vi "TestStand RunState Fields.vi"(2 "index":i32) -> (14 "Measurement Name":string, 15 "Low Limit":string, 16 "High Limit":string, 17 "Units":string, 18 "Comp":string, 19 "Data":string)   [LabVIEW 2010]
doc: "Creates strings with TestStand Numeric Test Property Names."
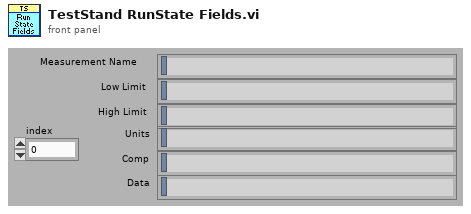
[diagram p1: front panel]
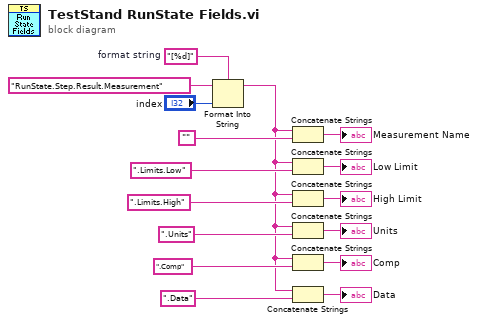
[diagram p0: block diagram]
diagram:
  w8 = "[%d]"  # format string
  n1 = Format Into String(format string=w8, initial string="RunState.Step.Result.Measurement" ("suffix"), "index") -> (resulting string=w1:string)  [unwired: 1 in, 1 out]
  n2 = Concatenate Strings(w1, "" ("prefix")) -> (→"Measurement Name":string)
  n3 = Concatenate Strings(w1, ".Limits.Low" ("prefix")) -> (→"Low Limit":string)
  n4 = Concatenate Strings(w1, ".Limits.High" ("prefix")) -> (→"High Limit":string)
  n5 = Concatenate Strings(w1, ".Units" ("prefix")) -> (→"Units":string)
  n6 = Concatenate Strings(w1, ".Comp" ("prefix")) -> (→"Comp":string)
  n7 = Concatenate Strings(w1, ".Data" ("prefix")) -> (→"Data":string)
